vi "SAVE SALE.vi"(11 "REFERENCES":T1) -> ()   [LabVIEW 2019]
uses:
  Controls/References Cluster.ctl
  <vilib>/userDefined/High Color/IMAQdx.ctl
  Controls/Custom Calendar/Custom Calendar.xctl
  Controls/Table Data Types/PSC Sales Data Type.ctl
  <vilib>/addons/database/Connection.llb/DB Tools Open Connec (String).vi
  <vilib>/addons/database/NI_Database_API.lvlib
types:
  T1 = typedef "References Cluster.ctl" = cluster{"MAIN PAGES":refnum<vi>, "ADD/EDIT ITEM REFERENCES":cluster{"Identifier":refnum<vi>, "BYU ICN #":refnum<vi>, "Item Description":refnum<vi>, "Comments":refnum<vi>, "Checked Out Date":refnum<vi>, "Due Date":refnum<vi>, "Check Out Location":refnum<vi>, "Reminder Count":refnum<vi>, "Most Recent Reminder Date":refnum<vi>, "BYU ID #":refnum<vi>, "Building/Room":refnum<vi>, "Location in Room":refnum<vi>, "Manual":refnum<vi>, "Manufacturer":refnum<vi>, "Model #":refnum<vi>, "Serial #":refnum<vi>, "Date Acquired":refnum<vi>, "ADD/EDIT ITEM LABEL":refnum<vi>, "ARCHIVE ITEM":refnum<vi>, "Archive Item Inputs":refnum<vi>, "Reminder Notes":refnum<vi>}, "ADD/EDIT USER REFERENCES":cluster{"BYU ID # (##-###-####)":refnum<vi>, "First Name":refnum<vi>, "Last Name":refnum<vi>, "Phone Number (###-###-####)":refnum<vi>, "Email":refnum<vi>, "Department":refnum<vi>, "Graduation Status":refnum<vi>, "Anticipated Graduation Year":refnum<vi>, "Credit Score":refnum<vi>, "Date Added":refnum<vi>, "Graduation Clearance Date":refnum<vi>, "Picture File Name":refnum<vi>, "ADD/EDIT USER LABEL":refnum<vi>, "Department Map":refnum<vi>, "Status Map":refnum<vi>, "Anticipated Graduation Year Map":refnum<vi>, "User Agreement":refnum<vi>, "User Comments":refnum<vi>, "Camera":refnum<vi>}, "RETURN ITEM REFERENCES":cluster{"Item or Person:":refnum<vi>, "Search Return Results":refnum<vi>, "What are you searching for?":refnum<vi>}, "SEARCH DATABASE REFERENCES":cluster{"What to Search For:":refnum<vi>, "Where to Search":refnum<vi>, "Column to Search In":refnum<vi>, "Column to Sort By":refnum<vi>, "Search Database Results":refnum<vi>, "Inventory Column Selector":refnum<vi>, "User Column Selector":refnum<vi>, "Inventory Archive Column Selector":refnum<vi>, "User Archive Column Selector":refnum<vi>, "Sales Tracking Column Selector":refnum<vi>, "Checked In Archive Column Selector":refnum<vi>, "Restore User":refnum<vi>, "Date Range":refnum<vi>, "Dates Less Than":refnum<vi>, "Dates Greater Than":refnum<vi>, "Search Print Receipt":refnum<vi>, "Edit Sale Description":refnum<vi>}, "USER ITEMS REFERENCES":cluster{"USER'S INFORMATION":refnum<vi>, "User's Checked Out Items":refnum<vi>, "User Info Comments":refnum<vi>, "SEE USER INFO COMMENTS":refnum<vi>}, "EDIT ITEMS REFERENCES":cluster{"New Check Out Location":refnum<vi>, "Items to Edit":refnum<vi>, "Edit Items Due Date":refnum<vi>, "New Reminder Notes":refnum<vi>, "New Item Description":refnum<vi>}, "CHECK OUT ITEMS REFERENCES":cluster{"Enter Item:":refnum<vi>, "Check Out Items Due Date":refnum<vi>, "Check Out Location":refnum<vi>, "Items to be Checked Out":refnum<vi>, "Possible Items":refnum<vi>, "Altered Item Description":refnum<vi>}, "TRANSFER ITEMS REFERENCES":cluster{"Search Parameter":refnum<vi>, "What to Match":refnum<vi>, "Matching Individuals":refnum<vi>, "Items to be Transferred":refnum<vi>}, "SETTINGS REFERENCES":cluster{"PSC Database Settings":refnum<vi>, "PSC Sales Item Spreadsheet":refnum<vi>}, "PSC SALES REFERENCES":cluster{"BYU ID CARD #":refnum<vi>, "Sale Description":refnum<vi>, "Scan or Enter Item Name":refnum<vi>, "Items to be Sold":refnum<vi>, "Grand Total":refnum<vi>, "Item List":refnum<vi>}}
  T2 = typedef "PSC Sales Data Type.ctl" = cluster{"SALE ID #":string, "BYU ID CARD #":string, "Sale Description":string, "Grand Total":string, "Sale Date":string, "Item Description":string, "Item Quantity":string, "Item Unit Price":string, "Item Total Price":string, "Sale Semester":string}
  T3 = cluster{"BYU ID CARD #":refnum<vi>, "Sale Description":refnum<vi>, "Scan or Enter Item Name":refnum<vi>, "Items to be Sold":refnum<vi>, "Grand Total":refnum<vi>, "Item List":refnum<vi>}
  T4 = typedef "NI_Database_API.lvlib/Conn ObjectReference.ctl" = refnum<k1>
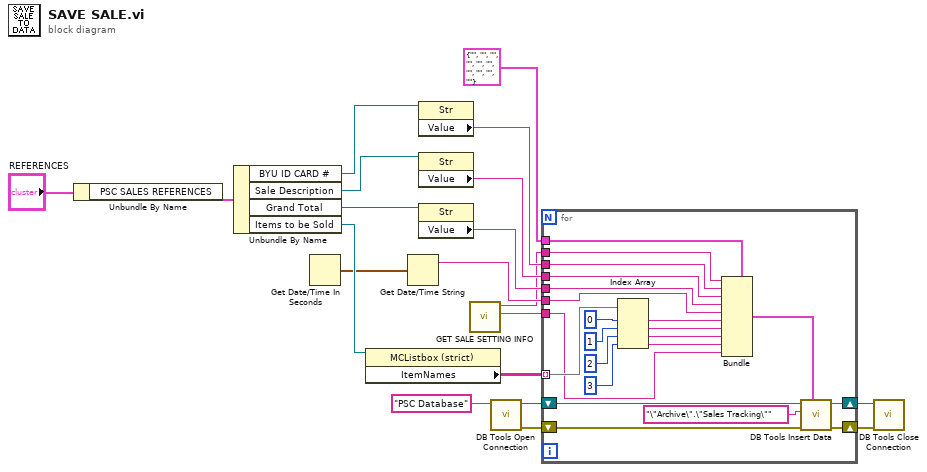
[diagram p0: block diagram]
diagram:
  n1 = Unbundle By Name("REFERENCES") -> ("PSC SALES REFERENCES"=w18:T3)
  n2 = Unbundle By Name(w18) -> ("BYU ID CARD #"=w17:refnum<vi>, "Sale Description"=w16:refnum<vi>, "Grand Total"=w15:refnum<vi>, "Items to be Sold"=w14:refnum<vi>)
  n3 = Get Date/Time In Seconds() -> (seconds since 1Jan1904=w4:timestamp)
  n4 = property class="MCListbox (strict)"(reference=w14) -> ("ItemNames"=w13:string[][])  [unwired: 1 in, 2 out]
  n5 = Get Date/Time String(seconds (now)=w4) -> (date string=w3:string)  [unwired: 2 in, 1 out]
  n6 = property class="Str"(reference=w17) -> ("Value"=w11:string)  [unwired: 1 in, 2 out]
  n7 = property class="Str"(reference=w16) -> ("Value"=w10:string)  [unwired: 1 in, 2 out]
  n8 = property class="Str"(reference=w15) -> ("Value"=w9:string)  [unwired: 1 in, 2 out]
  n9 = call "GET SALE SETTING INFO.vi"() -> ("Semester Out"=w1:string, "Identifier Out"=w2:string)  [unwired: 10 in]
  n10 = call-poly <vilib>:"DB Tools Open Connection.vi"("connection information"="PSC Database") -> ("error out"=w8:errorcluster, "connection reference"=w7:T4)  [unwired: 7 in]
  n11 = for {
    tunnel: w13 -> [w31] mode=indexing
    tunnel: T2 {"SALE ID #"="", "BYU ID CARD #"="", "Sale Description"="", "Grand Total"="", "Sale Date"="", "Item Description"="", "Item Quantity"="", "Item Unit Price"="", "Item Total Price"="", "Sale Semester"=""} ("PSC Sales Data Type") -> [w42]
    tunnel: w2 -> [w41]
    tunnel: w11 -> [w40]
    tunnel: w10 -> [w39]
    tunnel: w9 -> [w38]
    shift-right: [w33] -> w6
    shift-left: w7 -> [w34]
    shift-right: [w32] -> w5
    shift-left: w8 -> [w36]
    tunnel: w3 -> [w22]
    tunnel: w1 -> [w21]
    n12 = Index Array(array=w31, index #1=0 ("index"), index #2=1 ("index"), index #3=2 ("index"), index #4=3 ("index")) -> (element #1=w26:string, element #2=w25:string, element #3=w24:string, element #4=w23:string)
    n13 = Bundle(cluster=w42, "SALE ID #"=w41, "BYU ID CARD #"=w40, "Sale Description"=w39, "Grand Total"=w38, "Sale Date"=w22, "Item Description"=w26, "Item Quantity"=w25, "Item Unit Price"=w24, "Item Total Price"=w23, "Sale Semester"=w21) -> (w37:T2)
    n14 = call <vilib>:"DB Tools Insert Data.vi"("data"=w37, "error in (no error)"=w36, "table"="\"Archive\".\"Sales Tracking\"", "connection reference"=w34) -> ("error out"=w32:errorcluster, "connection reference out"=w33:T4)  [unwired: 6 in]
  }
  n15 = call <vilib>:"DB Tools Close Connection.vi"("error in (no error)"=w5, "connection reference"=w6) -> ()  [unwired: 5 in, 1 out]
